vi "Equal Unit Test.vi"(7 "String 2":string, 8 "entrée d'erreur (pas d'erreur)":errorcluster, 9 "String":string, 10 "Label":string, 11 "x+y":dbl) -> (0 "sortie d'erreur":errorcluster)   [LabVIEW 2021]
uses:
  <vilib>/addons/_JKI Toolkits/Caraya/classes/Properties.Assert/Properties.Assert.lvclass
  C:/Program Files (x86)/National Instruments/LabVIEW 2021/vi.lib/addons/_JKI Toolkits/Caraya/classes/Properties/Properties.lvclass
  <vilib>/addons/_JKI Toolkits/Caraya/classes/Assert/Assert Equal Value_Variant.vi
  <vilib>/addons/_JKI Toolkits/Caraya/classes/Assert/Assert.lvclass
  <vilib>/addons/_JKI Toolkits/Caraya/classes/Properties/Properties.lvclass
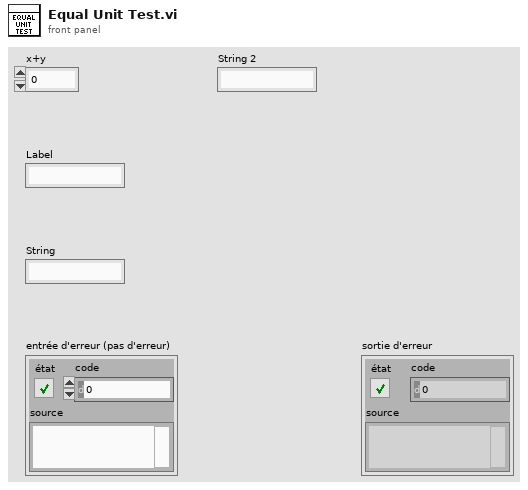
[diagram p1: front panel]
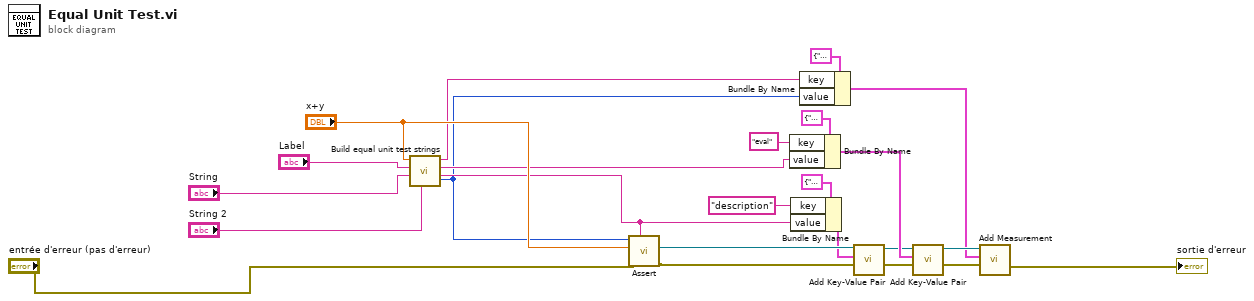
[diagram p0: block diagram]
diagram:
  n1 = call "Build equal unit test strings.vi"("String 2"="String 2", "String"="String", "Label"="Label", "x+y"="x+y") -> ("Chaîne 2"=w19:string, "Chaîne"=w22:string, "Chaîne 3"=w18:string, "Numérique"=w15:i32)  [unwired: 4 in]
  n2 = call-poly <vilib>:"Assert.vi"("Label"=w19, "error in (no error)"="entrée d'erreur (pas d'erreur)", "Y"="x+y", "X"=w15) -> ("error out"=w14:errorcluster, "Properties.Assert"=w16:refnum<class "Properties.Assert.lvclass">)  [unwired: 6 in]
  n3 = Bundle By Name(cluster=cluster{"key":string, "value":variant} {"key"="", "value"=variant} ("entry"), "key"="eval", "value"=w22) -> (w12:cluster{"key":string, "value":variant})
  n4 = Bundle By Name(cluster=cluster{"key":string, "value":variant} {"key"="", "value"=variant} ("entry"), "key"="description", "value"=w19) -> (w3:cluster{"key":string, "value":variant})
  n5 = Bundle By Name(cluster=cluster{"key":string, "value":variant} {"key"="", "value"=variant} ("entry"), "key"=w18, "value"=w15) -> (w6:cluster{"key":string, "value":variant})
  n6 = call <vilib>:"Add Key-Value Pair.vi"("error in (no error)"=w14, "entry"=w3, "Properties in"=w16) -> ("error out"=w7:errorcluster, "Properties out"=w9:refnum<class "Properties.Assert.lvclass">)  [unwired: 7 in]
  n7 = call <vilib>:"Add Key-Value Pair.vi"("error in (no error)"=w7, "entry"=w12, "Properties in"=w9) -> ("error out"=w8:errorcluster, "Properties out"=w10:refnum<class "Properties.Assert.lvclass">)  [unwired: 7 in]
  n8 = call <vilib>:"Add Measurement.vi"("error in (no error)"=w8, "entry"=w6, "Properties"=w10) -> ("error out"=→"sortie d'erreur":errorcluster)  [unwired: 7 in, 1 out]
